vi "GP1 get pressure.vi"(3 "error in":errorcluster) -> (0 "error out":errorcluster, 1 "Baratron (Torr)":dbl, 2 "Actual (psi)":dbl)   [LabVIEW 2020, in "GP1.lvclass"]
uses:
  GP1.lvclass
  DAQmx Read (Analog DBL 1Chan 1Samp).vi
  DAQmx Read (Analog 1D DBL 1Chan NSamp).vi
  Mean (DBL).vi
  DAQmx Fill In Error Info.vi
  NI_AALBase.lvlib
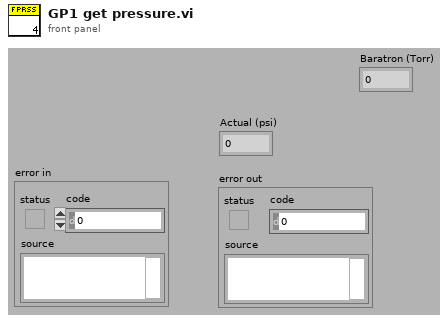
[diagram p1: front panel]
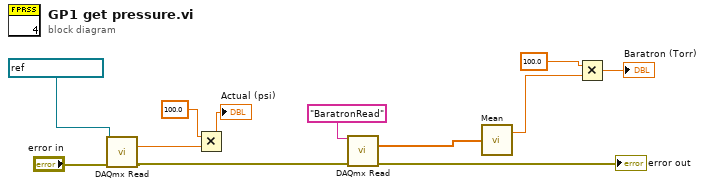
[diagram p0: block diagram]
diagram:
  n1 = call-poly "DAQmx Read.vi"("task/channels in"=refnum<k21> "pressureread" ("readtask"), "error in"="error in") -> ("data"=w11:dbl, "error out"=w6:errorcluster)  [unwired: 12 out]
  n2 = Multiply(x=100.0 ("y"), y=w11) -> (x*y=→"Actual (psi)":dbl)
  n3 = call-poly "DAQmx Read.vi"("task/channels in"="BaratronRead" ("new task name"), "error in"=w6) -> ("data"=w4:dbl[], "error out"=→"error out":errorcluster)  [unwired: 2 in, 10 out]
  n4 = call-poly "Mean.vi"("X"=w4) -> ("mean"=w2:dbl)  [unwired: 1 out]
  n5 = Multiply(x=100.0 ("y"), y=w2) -> (x*y=→"Baratron (Torr)":dbl)
